vi "Open Handle.vi"(6 "verify server (T)":bool=TRUE, 7 "cookie file":path, 8 "error in (no error)":errorcluster, 9 "password":string, 10 "username":string, 11 "HTTP Client Advanced in":refnum<class "HTTP Client Advanced.lvclass">) -> (0 "error out":errorcluster, 3 "HTTP Client Advanced out":refnum<class "HTTP Client Advanced.lvclass">)   [LabVIEW 2021, in "HTTP Client Advanced.lvclass"]
uses:
  HTTP Client Advanced.lvclass
  HTTP Client Advanced.lvclass/HTTP Client Advanced.ctl
  <vilib>/NI/Advanced HTTP Client/Session.lvclass
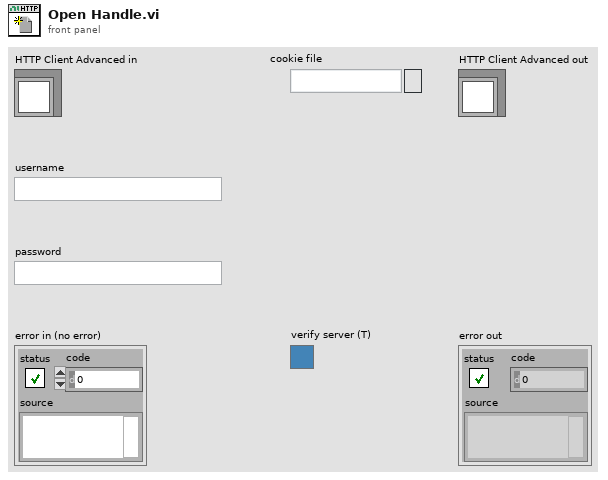
[diagram p1: front panel]
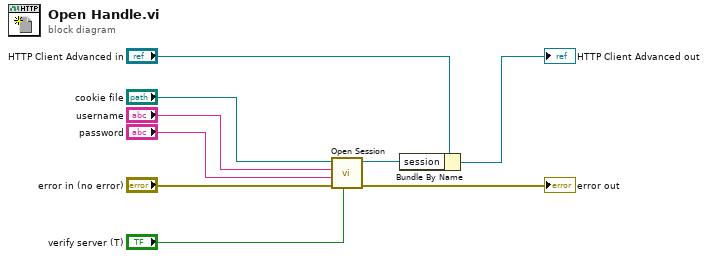
[diagram p0: block diagram]
diagram:
  n1 = call <vilib>:"Open Session.vi"("verify server (T)"="verify server (T)", "error in"="error in (no error)", "password"="password", "username"="username", "cookie file"="cookie file") -> ("error out"=→"error out":errorcluster, "session"=w2:refnum<class "Session.lvclass">)  [unwired: 5 in]
  n2 = Bundle By Name(cluster="HTTP Client Advanced in", "session"=w2) -> (→"HTTP Client Advanced out":refnum<class "HTTP Client Advanced.lvclass">)
